vi "CONFIRM SELECTION.vi"(11 "REFERENCES":T2) -> (3 "STATE OUT":T1)   [LabVIEW 2019]
uses:
  Controls/References Cluster.ctl
  Controls/Custom Calendar/Custom Calendar.xctl
  Controls/State Variables/Transfer Items States.ctl
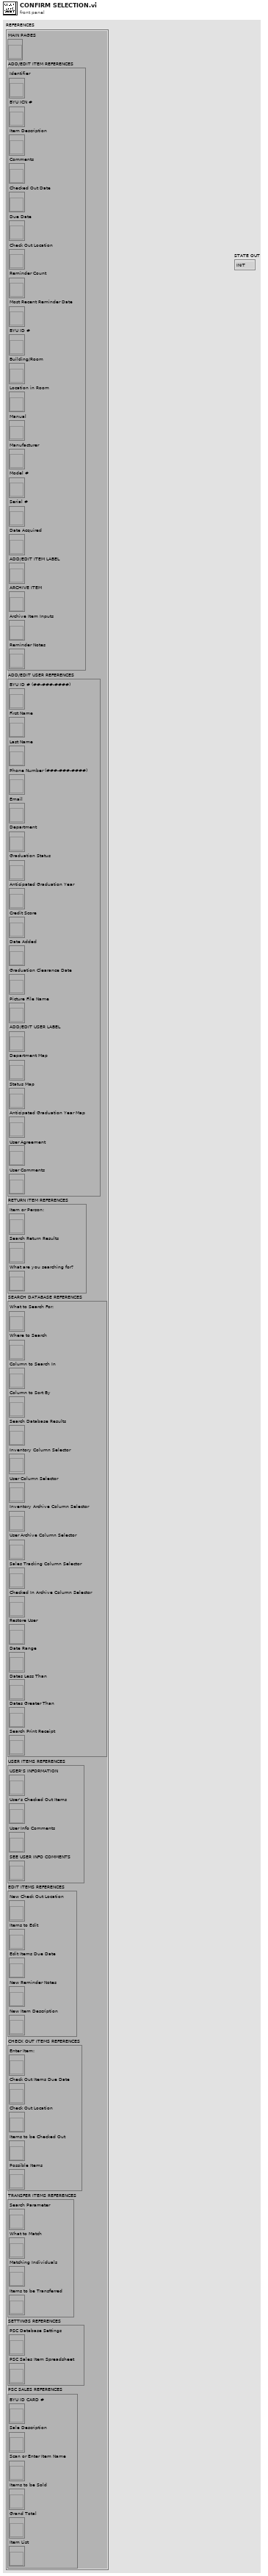
[diagram p1: front panel]
types:
  T1 = typedef "Transfer Items States.ctl" = enum16{"INIT", "IDLE", "FIND USER", "CONFIRM SELECTION", "REMOVE ITEMS", "TRANSFER ITEMS", "END"}
  T2 = typedef "References Cluster.ctl" = cluster{"MAIN PAGES":refnum<vi>, "ADD/EDIT ITEM REFERENCES":cluster{"Identifier":refnum<vi>, "BYU ICN #":refnum<vi>, "Item Description":refnum<vi>, "Comments":refnum<vi>, "Checked Out Date":refnum<vi>, "Due Date":refnum<vi>, "Check Out Location":refnum<vi>, "Reminder Count":refnum<vi>, "Most Recent Reminder Date":refnum<vi>, "BYU ID #":refnum<vi>, "Building/Room":refnum<vi>, "Location in Room":refnum<vi>, "Manual":refnum<vi>, "Manufacturer":refnum<vi>, "Model #":refnum<vi>, "Serial #":refnum<vi>, "Date Acquired":refnum<vi>, "ADD/EDIT ITEM LABEL":refnum<vi>, "ARCHIVE ITEM":refnum<vi>, "Archive Item Inputs":refnum<vi>, "Reminder Notes":refnum<vi>}, "ADD/EDIT USER REFERENCES":cluster{"BYU ID # (##-###-####)":refnum<vi>, "First Name":refnum<vi>, "Last Name":refnum<vi>, "Phone Number (###-###-####)":refnum<vi>, "Email":refnum<vi>, "Department":refnum<vi>, "Graduation Status":refnum<vi>, "Anticipated Graduation Year":refnum<vi>, "Credit Score":refnum<vi>, "Date Added":refnum<vi>, "Graduation Clearance Date":refnum<vi>, "Picture File Name":refnum<vi>, "ADD/EDIT USER LABEL":refnum<vi>, "Department Map":refnum<vi>, "Status Map":refnum<vi>, "Anticipated Graduation Year Map":refnum<vi>, "User Agreement":refnum<vi>, "User Comments":refnum<vi>}, "RETURN ITEM REFERENCES":cluster{"Item or Person:":refnum<vi>, "Search Return Results":refnum<vi>, "What are you searching for?":refnum<vi>}, "SEARCH DATABASE REFERENCES":cluster{"What to Search For:":refnum<vi>, "Where to Search":refnum<vi>, "Column to Search In":refnum<vi>, "Column to Sort By":refnum<vi>, "Search Database Results":refnum<vi>, "Inventory Column Selector":refnum<vi>, "User Column Selector":refnum<vi>, "Inventory Archive Column Selector":refnum<vi>, "User Archive Column Selector":refnum<vi>, "Sales Tracking Column Selector":refnum<vi>, "Checked In Archive Column Selector":refnum<vi>, "Restore User":refnum<vi>, "Date Range":refnum<vi>, "Dates Less Than":refnum<vi>, "Dates Greater Than":refnum<vi>, "Search Print Receipt":refnum<vi>}, "USER ITEMS REFERENCES":cluster{"USER'S INFORMATION":refnum<vi>, "User's Checked Out Items":refnum<vi>, "User Info Comments":refnum<vi>, "SEE USER INFO COMMENTS":refnum<vi>}, "EDIT ITEMS REFERENCES":cluster{"New Check Out Location":refnum<vi>, "Items to Edit":refnum<vi>, "Edit Items Due Date":refnum<vi>, "New Reminder Notes":refnum<vi>, "New Item Description":refnum<vi>}, "CHECK OUT ITEMS REFERENCES":cluster{"Enter Item:":refnum<vi>, "Check Out Items Due Date":refnum<vi>, "Check Out Location":refnum<vi>, "Items to be Checked Out":refnum<vi>, "Possible Items":refnum<vi>}, "TRANSFER ITEMS REFERENCES":cluster{"Search Parameter":refnum<vi>, "What to Match":refnum<vi>, "Matching Individuals":refnum<vi>, "Items to be Transferred":refnum<vi>}, "SETTINGS REFERENCES":cluster{"PSC Database Settings":refnum<vi>, "PSC Sales Item Spreadsheet":refnum<vi>}, "PSC SALES REFERENCES":cluster{"BYU ID CARD #":refnum<vi>, "Sale Description":refnum<vi>, "Scan or Enter Item Name":refnum<vi>, "Items to be Sold":refnum<vi>, "Grand Total":refnum<vi>, "Item List":refnum<vi>}}
  T3 = cluster{"Search Parameter":refnum<vi>, "What to Match":refnum<vi>, "Matching Individuals":refnum<vi>, "Items to be Transferred":refnum<vi>}
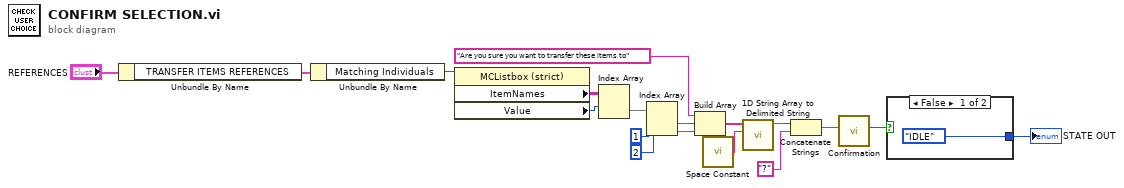
[diagram p0: block diagram]
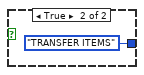
[diagram p2: hidden frame]
diagram:
  n1 = Unbundle By Name("REFERENCES") -> ("TRANSFER ITEMS REFERENCES"=w17:T3)
  n2 = Unbundle By Name(w17) -> ("Matching Individuals"=w16:refnum<vi>)
  n3 = property class="MCListbox (strict)"(reference=w16) -> ("ItemNames"=w15:string[][], "Value"=w1:i32)  [unwired: 1 in, 2 out]
  n4 = Index Array(array=w15, index (row)=w1) -> (element=w14:string[])  [unwired: 1 in]
  n5 = Index Array(array=w14, index #1=1 ("index"), index #2=2 ("index")) -> (element #1=w10:string, element #2=w9:string)
  n6 = Build Array("Are you sure you want to transfer these items to" ("string"), w10, w9) -> (w8:string[])
  n7 = call <vilib>:"Space Constant.vi"() -> ("String"=w7:string)
  n8 = call <vilib>:"1D String Array to Delimited String.vi"("delimiter"=w7, "string array"=w8) -> ("delimited string"=w6:string)  [unwired: 9 in]
  n9 = Concatenate Strings(w6, "?" ("string")) -> (w4:string)
  n10 = call "Confirmation"("Message"=w4) -> ("YES"=w3:bool)  [unwired: 9 in, 1 out]
  n11 = case shown="False" w3 {
    tunnel: [Transfer_Items_States."IDLE" Transfer_Items_States."TRANSFER ITEMS"] -> w2
    frame False {
    }
    frame True {
    }
  }
  "STATE OUT" <- w2
